vi "GetConductanceIntensity.vi"(7 "LabVIEW Web Service Request":refnum<class "Web Request.lvclass">) -> ()   [LabVIEW 2016]
uses:
  <vilib>/wsapi/Web Request.lvclass
  <vilib>/wsapi/NI_WebServices.lvlib
panel:
  # "Use the Web Service Request input terminal to call the VIs on the Web Services palette. Do not remove it from the connector pane unless you don't need access to the palette."
  # "Each additional control wired to the connector pane will be available as an input in the URL. To include an indicator in terminal-mode output (the default setting), it must also be wired to the connector pane."
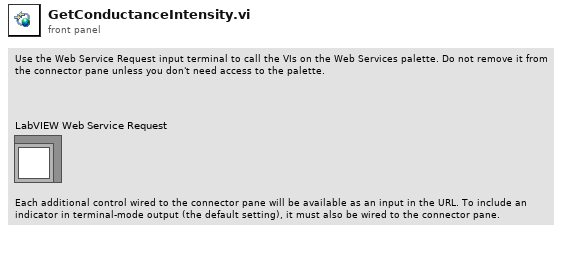
[diagram p1: front panel]
types:
  T1 = typedef "imagedata.ctl" = cluster{"image type":i32, "image depth":i32, "image":u8[], "mask":u8[], "colors":u32[], "Rectangle":cluster{"left":i16, "top":i16, "right":i16, "bottom":i16}}
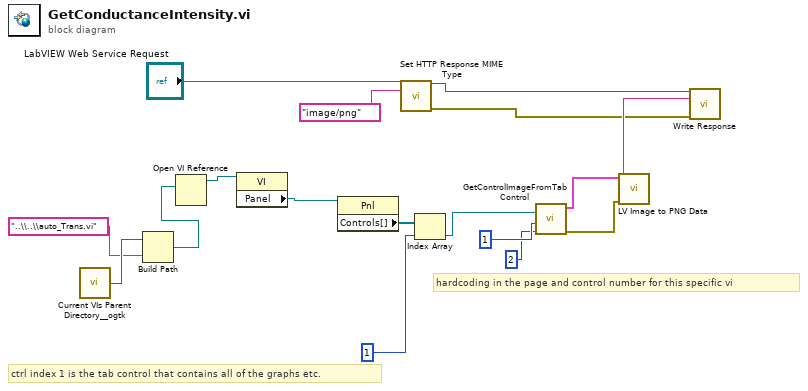
[diagram p0: block diagram]
diagram:
  # "hardcoding in the page and control number for this specific vi"
  # "ctrl index 1 is the tab control that contains all of the graphs etc."
  n1 = call <userlib>:"Current VIs Parent Directory__ogtk.vi"() -> ("Parent Directory (+ Relative)"=w12:path)  [unwired: 5 in]
  n2 = Build Path(base path=w12, name or relative path="..\\..\\auto_Trans.vi") -> (appended path=w10:path)
  n3 = Open VI Reference(vi path=w10) -> (vi reference=w13:refnum<vi>)  [unwired: 5 in, 1 out]
  n4 = property class="VI"(reference=w13) -> ("Panel"=w9:refnum<vi>)  [unwired: 1 in, 2 out]
  n5 = property class="Pnl"(reference=w9) -> ("Controls[]"=w8:refnum<vi>[])  [unwired: 1 in, 2 out]
  n6 = call <vilib>:"Set HTTP Response MIME Type.vi"("LabVIEW Web Service Request"="LabVIEW Web Service Request", "MIME type (text/html)"="image/png") -> ("LabVIEW Web Service Request out"=w16:refnum<class "Web Request.lvclass">, "error out"=w14:errorcluster)  [unwired: 12 in]
  n7 = Index Array(array=w8, index=1) -> (element=w5:refnum<vi>)
  n8 = call "GetControlImageFromTabControl.vi"("page"=2, "control"=1, "Ctl Refnum"=w5) -> ("error out"=w3:errorcluster, "image data"=w4:T1)  [unwired: 6 in, 1 out]
  n9 = call <vilib>:"LV Image to PNG Data.vi"("error in (no error)"=w3, "image data"=w4) -> ("png data"=w15:string)  [unwired: 8 in, 1 out]
  n10 = call <vilib>:"Write Response.vi"("LabVIEW Web Service Request"=w16, "response string"=w15, "error in (no error)"=w14) -> ()  [unwired: 11 in, 2 out]
